vi "Close Device.vi"(8 "error in (no error)":errorcluster, 11 "NI DAQmx in":refnum<class "NI DAQmx.lvclass">) -> (0 "error out":errorcluster, 3 "NI DAQmx out":refnum<class "NI DAQmx.lvclass">)   [LabVIEW 2020, in "NI DAQmx.lvclass"]
uses:
  NI DAQmx.lvclass
  <vilib>/DAQmx/write.llb/DAQmx Write (Digital Bool 1Line 1Point).vi
  <vilib>/DAQmx/miscellaneous.llb/DAQmx Fill In Error Info.vi
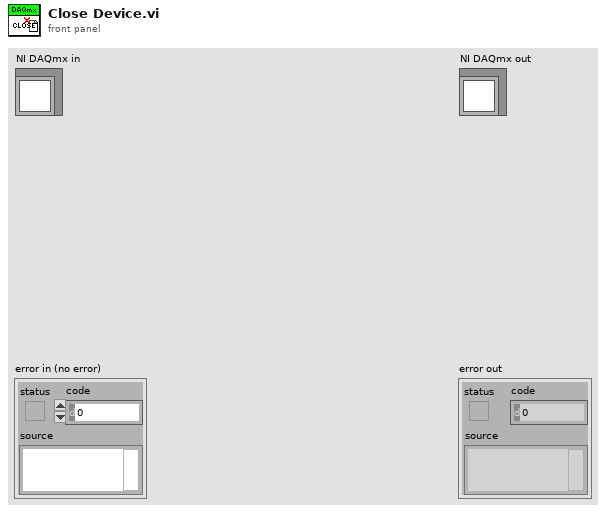
[diagram p1: front panel]
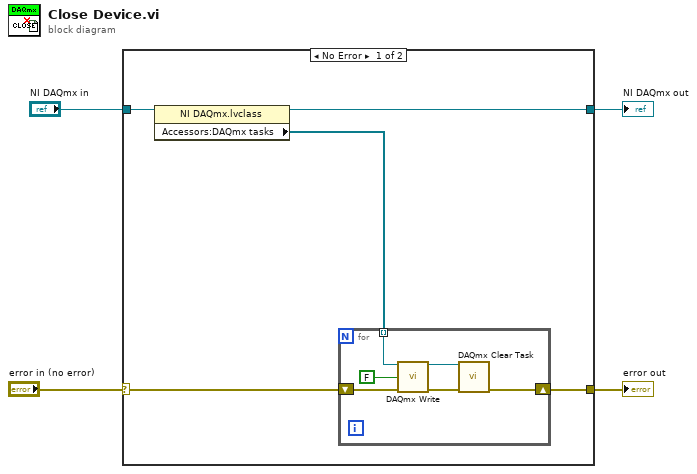
[diagram p0: block diagram]
diagram:
  n1 = case shown="No Error" "error in (no error)" {
    selector: "error in (no error)" -> [w7 w17]
    tunnel: [w6 w17] -> w3
    tunnel: [w5 w16] -> w2
    tunnel: "NI DAQmx in" -> [w9 w16]
    frame No Error {
      n2 = property class="NI DAQmx.lvclass"(reference=w9) -> (reference out=w5:refnum<class "NI DAQmx.lvclass">, "Accessors:DAQmx tasks"=w8:refnum<k21>[])  [unwired: 1 in, 1 out]
      n3 = for {
        tunnel: w8 -> [w11] mode=indexing
        shift-right: [w15] -> w6
        shift-left: w7 -> [w14]
        n4 = call-poly <vilib>:"DAQmx Write.vi"("task/channels in"=w11, "data"=FALSE, "error in"=w14) -> ("task out"=w12:refnum<k21>, "error out"=w13:errorcluster)  [unwired: 10 in, 1 out]
        n5 = call <vilib>:"DAQmx Clear Task.vi"("task in"=w12, "error in"=w13) -> ("error out"=w15:errorcluster)  [unwired: 13 in]
      }
    }
    frame Error {
    }
  }
  "error out" <- w3
  "NI DAQmx out" <- w2
